vi "totorial-066.vi"() -> ()   [LabVIEW 2021]
uses:
  TextControlledInstrum/ControlToCommandMulti.vi
  TextControlledInstrum/TextControlledInstrum.lvlib
panel:
  in  "C":string
  in  "B":cluster{"B1":dbl, "B2":dbl}
  in  "A":dbl
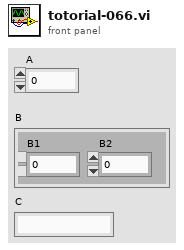
[diagram p1: front panel]
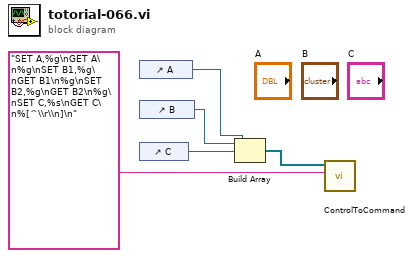
[diagram p0: block diagram]
diagram:
  n1 = control-ref of="A"() -> (w5:refnum<vi>)
  n2 = control-ref of="B"() -> (w4:refnum<vi>)
  n3 = control-ref of="C"() -> (w3:refnum<vi>)
  n4 = Build Array(w5, w4, w3) -> (w2:refnum<vi>[])
  n5 = call-poly "ControlToCommand.vi"("SetGetCommands"="SET A,%g\nGET A\n%g\nSET B1,%g\nGET B1\n%g\nSET B2,%g\nGET B2\n%g\nSET C,%s\nGET C\n%[^\\r\\n]\n", "Control Array"=w2) -> ()  [unwired: 9 in, 1 out]
